vi "Wait for Data.vi"(0 "Wait Notifier":refnum<notifier>, 11 "Error In":errorcluster) -> (8 "Data":variant, 15 "Error Out":errorcluster)   [LabVIEW 2023, in "Message Handler.lvclass"]
uses:
  Message Handler.lvclass
  Message Handler.lvclass/Message Handler.ctl
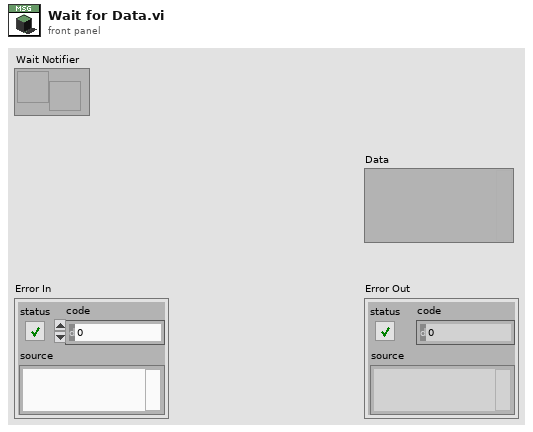
[diagram p1: front panel]
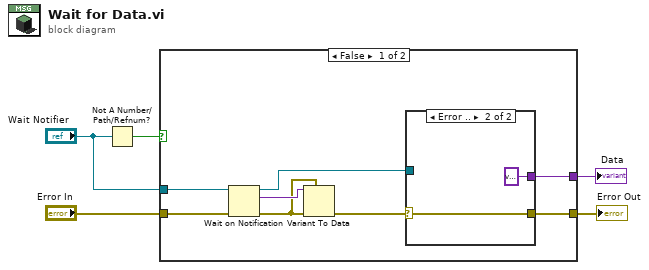
[diagram p0: block diagram]
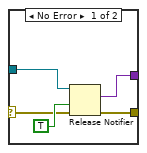
[diagram p2: hidden frame]
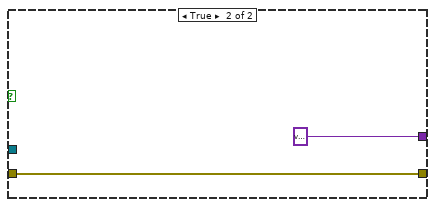
[diagram p3: hidden frame]
diagram:
  n1 = Not A Number/Path/Refnum?(number/path/refnum="Wait Notifier") -> (NaN/Path/Refnum?=w5:bool)
  n2 = case shown="False" w5 {
    tunnel: [w9 variant ("element data type")] -> w4
    tunnel: "Wait Notifier" -> [w13 _]
    tunnel: "Error In" -> [w12 w21]
    tunnel: [w10 w21] -> w1
    frame False {
      n3 = Wait on Notification(notifier=w13, error in (no error)=w12) -> (notifier out=w11:refnum<notifier>, notification=w8:variant, error out=w7:errorcluster)  [unwired: 2 in, 1 out]
      n4 = Variant To Data(error in=w7, type=w7, Variant=w8) -> (error out=w6:errorcluster)  [unwired: 1 out]
      n5 = case shown="Error .." w6 {
        selector: w6 -> [w14 w19]
        tunnel: w11 -> [w18 _]
        tunnel: [w17 w19] -> w10
        tunnel: [w16 variant ("element data type")] -> w9
        frame No Error {
          n6 = Release Notifier(notifier=w18, force destroy? (F)=TRUE, error in (no error)=w14) -> (last notification=w16:variant, error out=w17:errorcluster)  [unwired: 1 out]
        }
        frame Error {
        }
      }
    }
    frame True {
    }
  }
  "Error Out" <- w1
  "Data" <- w4
